vi "Write_Alarm_State.vi"(8 "error in (no error)":errorcluster, 9 "Alarm_State":bool=TRUE, 11 "MHL_Data In":T1) -> (0 "error out":errorcluster, 3 "MHL_Data Out":T1)   [LabVIEW 2019, in "MHL.lvlib"]
uses:
  MHL.lvlib
  typedef/MHL_Data.ctl
  Alarm_Panel/Channel_Temperature_Threshold.ctl
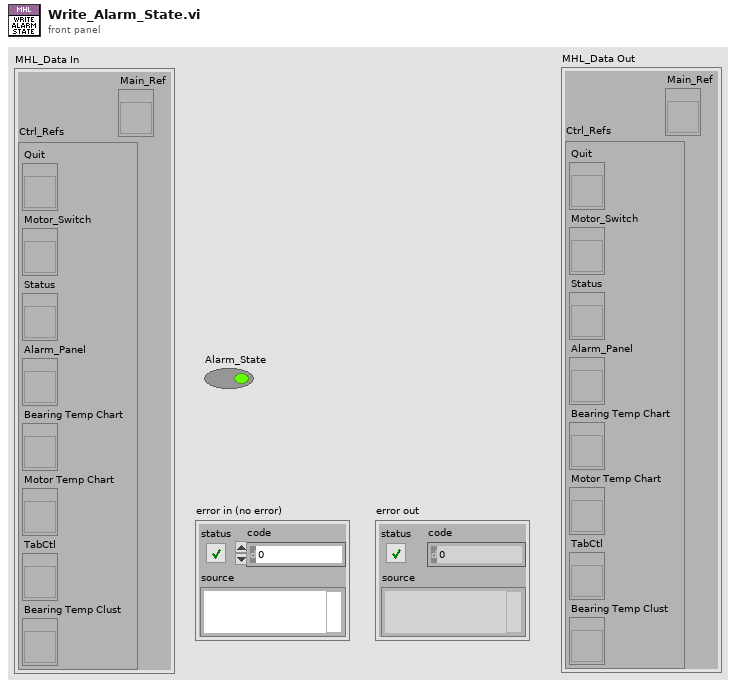
[diagram p1: front panel]
types:
  T1 = typedef "MHL.lvlib/MHL_Data.ctl" = cluster{"Ctrl_Refs":cluster{"Quit":refnum<vi>, "Motor_Switch":refnum<vi>, "Status":refnum<vi>, "Alarm_Panel":refnum<vi>, "Bearing Temp Chart":refnum<vi>, "Motor Temp Chart":refnum<vi>, "TabCtl":refnum<vi>, "Bearing Temp Clust":refnum<vi>}, "Main_Ref":refnum<vi>}
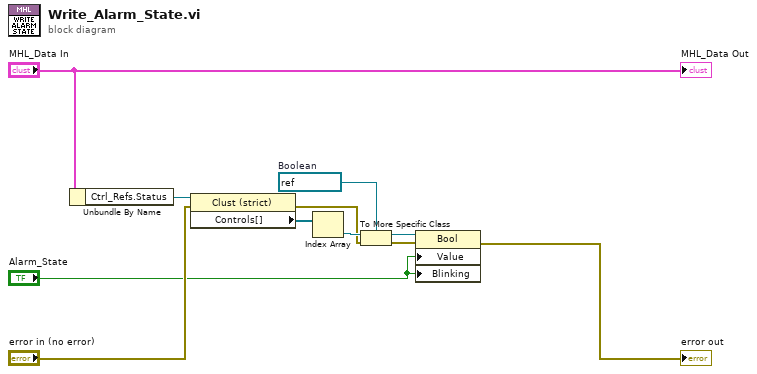
[diagram p0: block diagram]
diagram:
  w7 = refnum<vi> refnum  # Boolean
  n1 = Unbundle By Name("MHL_Data In") -> ("Ctrl_Refs.Status"=w11:refnum<vi>)
  n2 = property class="Clust (strict)"(reference=w11, error in="error in (no error)") -> (error out=w5:errorcluster, "Controls[]"=w9:refnum<vi>[])  [unwired: 1 out]
  n3 = Index Array(array=w9) -> (element=w8:refnum<vi>)  [unwired: 1 in]
  n4 = To More Specific Class(target class=w7, reference=w8, error in=w5) -> (specific class reference=w6:refnum<vi>, error out=w4:errorcluster)
  n5 = property class="Bool"(reference=w6, error in=w4, "Value"="Alarm_State", "Blinking"="Alarm_State") -> (error out=→"error out":errorcluster)  [unwired: 1 out]
  "MHL_Data Out" <- "MHL_Data In"
